vi "Boolean to Disabled Enum.vi"(1 "Grey Out (T)":bool=TRUE, 2 "Enable":bool) -> (0 "Disabled":T1(ring))   [LabVIEW 2023, in "Utilities.lvlib"]
uses:
  Utilities.lvlib
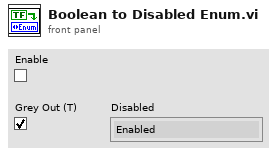
[diagram p1: front panel]
types:
  T1 = enum8{"Enabled", "Disabled", "Disabled and Grayed Out"}
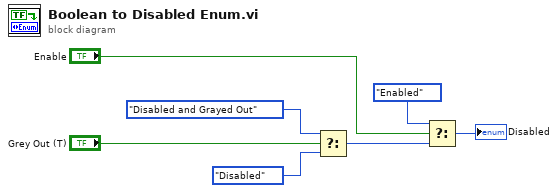
[diagram p0: block diagram]
diagram:
  n1 = Select(t=T1."Disabled and Grayed Out" ("Disabled"), s="Grey Out (T)", f=T1."Disabled" ("Disabled")) -> (s? t:f=w3:T1)
  n2 = Select(t=T1."Enabled" ("Disabled"), s="Enable", f=w3) -> (s? t:f=→"Disabled":T1)
